vi "Determine Clicked Array Element Index - Determine Array and Scrollbar Properties.vi"(8 "error in (no error)":errorcluster, 10 "Coords of Click":T1, 11 "Array Reference":refnum<vi>) -> (0 "error out":errorcluster, 1 "Scrollbar Properties":T2, 2 "Array Properties":T5, 3 "dup Array Reference":refnum<vi>)   [LabVIEW 2016]
doc: "Determine Clicked Array Element Index - Determine Array and Scrollbar Properties.vi\n\nDescription:\nThis VI determines multiple properties of the array and scrollbars of the array specified by the Array Reference input.\n\nIf no caption has been created for the array of interest, instruct the user how to correct the issue.\n\nInputs:\nArray Reference - Reference to the array to operate on.\n\nCoords of Click - The screen coordinates of the click within the array. These values are used to determine if the click occurred on the selected item.\n\nerror in - Standard error cluster.\n\nOutputs:\ndup Array Reference - Dup reference to the array to operate on.\n\nArray Properties - Cluster containing the array properties of the array specified by the Array Reference input.\n\nScrollbar Properties - Cluster containing the scrollbar properties of the array specified by the Array Reference input.\n\nerror out - standard error cluster.\n\nDeveloped By:\nMark.ridgley\nMark.Ridgley_LabVIEW.Developer@comcast.net"
uses:
  <vilib>/Utility/miscctls.llb/LVBoundsTypeDef.ctl
  <vilib>/Utility/miscctls.llb/LVPositionTypeDef.ctl
  <vilib>/Utility/miscctls.llb/LVPoint32TypeDef.ctl
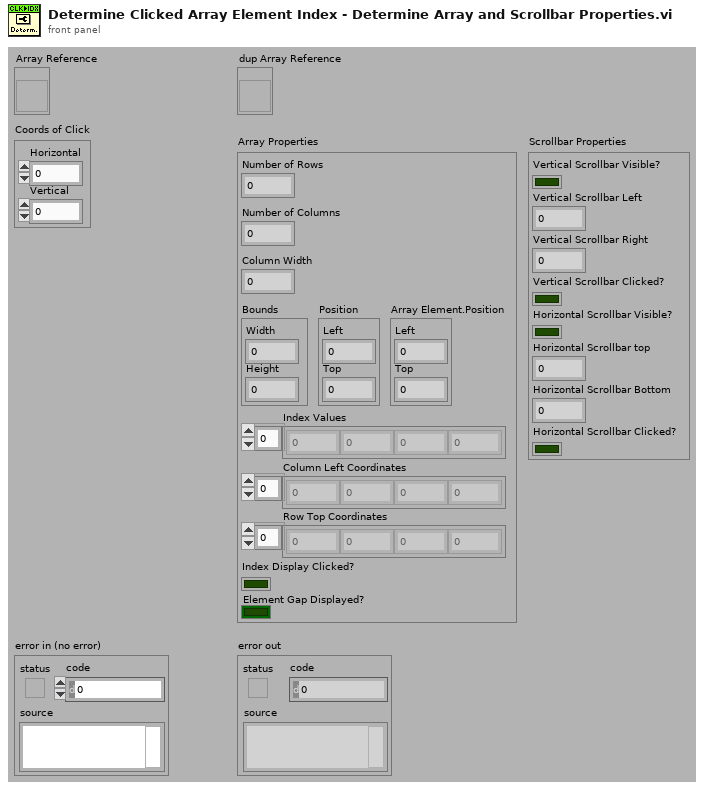
[diagram p1: front panel]
types:
  T1 = typedef "LVPoint32TypeDef.ctl" = cluster{"Horizontal":i32, "Vertical":i32}
  T2 = cluster{"Vertical Scrollbar Visible?":bool, "Vertical Scrollbar Left":i32, "Vertical Scrollbar Right":i32, "Vertical Scrollbar Clicked?":bool, "Horizontal Scrollbar Visible? ":bool, "Horizontal Scrollbar top":i32, "Horizontal Scrollbar Bottom":i32, "Horizontal Scrollbar Clicked?":bool}
  T3 = typedef "LVBoundsTypeDef.ctl" = cluster{"Width":u32, "Height":u32}
  T4 = typedef "LVPositionTypeDef.ctl" = cluster{"Left":i32, "Top":i32}
  T5 = cluster{"Number of Rows":u32, "Number of Columns":u32, "Column Width":u32, "Bounds":T3, "Position":T4, "Array Element.Position":T4, "Index Values":u32[], "Column Left Coordinates":i32[], "Row Top Coordinates":i32[], "Index Display Clicked?":bool, "Element Gap Displayed?":bool}
  T6 = enum16{"Horizontal Scrollbar", "Vertical Scrollbar"}
  T7 = enum16{"Horizontal Scrollbar", "Vertical Scrollbar", "Index Display"}
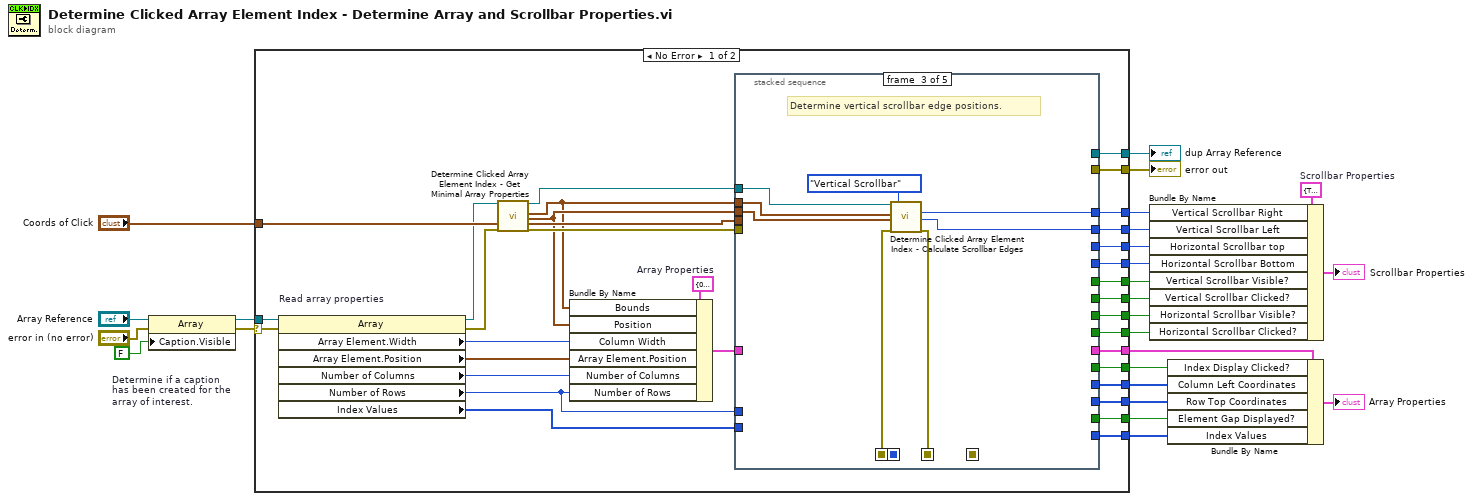
[diagram p0: block diagram]
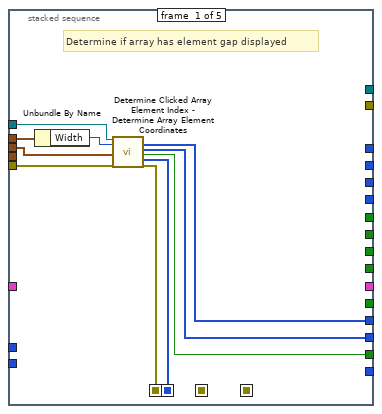
[diagram p2: hidden frame]
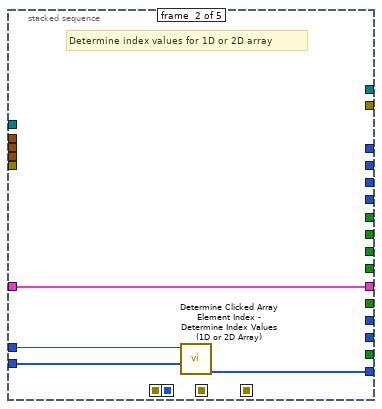
[diagram p3: hidden frame]
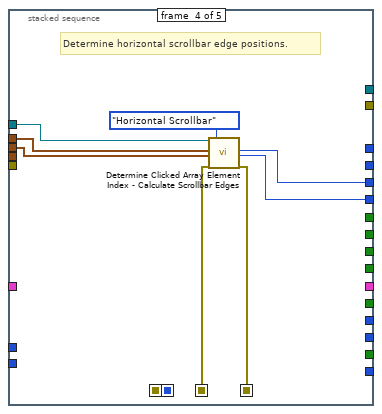
[diagram p4: hidden frame]
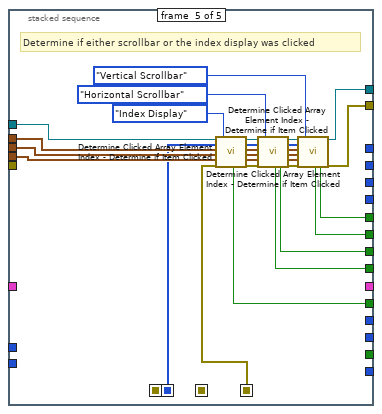
[diagram p5: hidden frame]
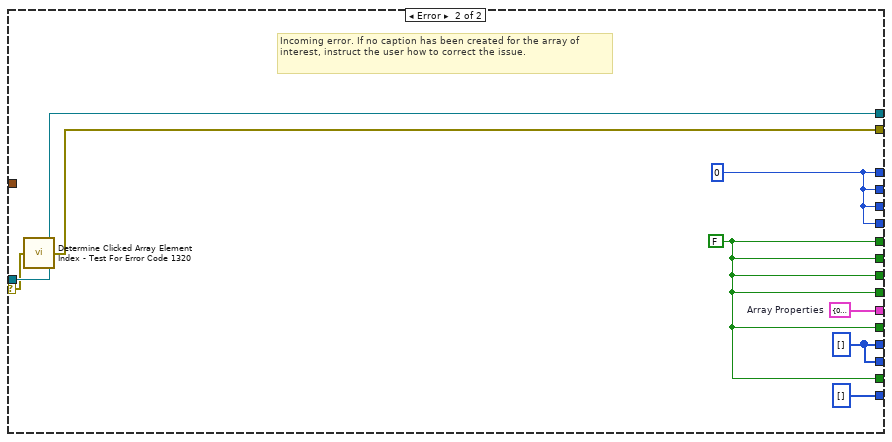
[diagram p6: hidden frame]
diagram:
  w1 = T2 {"Vertical Scrollbar Visible?"=TRUE, "Vertical Scrollbar Left"=0, "Vertical Scrollbar Right"=0, "Vertical Scrollbar Clicked?"=FALSE, "Horizontal Scrollbar Visible? "=TRUE, "Horizontal Scrollbar top"=0, "Horizontal Scrollbar Bottom"=0, "Horizontal Scrollbar Clicked?"=TRUE}  # Scrollbar Properties
  n1 = property on="Determine if a caption has been created for the array of interest." class="Array"(reference="Array Reference", error in="error in (no error)", "Caption.Visible"=FALSE) -> (reference out=w6:refnum<vi>, error out=w7:errorcluster)
  n2 = case shown="No Error" w7 {
    selector: w7 -> [w30 w121]
    tunnel: "Coords of Click" -> [w58 _]
    tunnel: [w57 u32[] [] ("Column Left Coordinates")] -> w23
    tunnel: w6 -> [w56 w124]
    tunnel: [w53 w123] -> w22
    tunnel: [w52 w123] -> w21
    tunnel: [w51 w123] -> w20
    tunnel: [w50 w123] -> w19
    tunnel: [w49 w123] -> w18
    tunnel: [w46 w124] -> w17
    tunnel: [w45 w117] -> w16
    tunnel: [w44 w117] -> w15
    tunnel: [w42 w122] -> w14
    tunnel: [w41 w122] -> w13
    tunnel: [w40 w123] -> w12
    tunnel: [w32 w118] -> w11
    tunnel: [w31 w120] -> w10
    tunnel: [w27 w117] -> w3
    tunnel: [w26 w117] -> w2
    frame No Error {
      w28 = T5 {"Number of Rows"=0, "Number of Columns"=0, "Column Width"=0, "Bounds"={"Width"=0, "Height"=0}, "Position"={"Left"=0, "Top"=0}, "Array Element.Position"={"Left"=0, "Top"=0}, "Index Values"=[], "Column Left Coordinates"=[], "Row Top Coordinates"=[], "Index Display Clicked?"=FALSE, "Element Gap Displayed?"=FALSE}  # Array Properties
      n3 = property on="Read array properties" class="Array"(reference=w56, error in=w30) -> (reference out=w54:refnum<vi>, error out=w55:errorcluster, "Array Element.Width"=w29:u32, "Array Element.Position"=w36:T4, "Number of Columns"=w34:u32, "Number of Rows"=w35:u32, "Index Values"=w37:u32[])
      n4 = call "Determine Clicked Array Element Index - Get Minimal Array Properties.vi"("Array Reference"=w54, "Coords of Click"=w58, "error in (no error)"=w55) -> ("dup Array Reference"=w43:refnum<vi>, "Minimal Array Properties.Bounds"=w38:T3, "Minimal Array Properties.Position"=w39:T4, "dup Coords of Click"=w48:T1, "error out"=w47:errorcluster)  [unwired: 12 in]
      n5 = Bundle By Name(cluster=w28, "Bounds"=w38, "Position"=w39, "Column Width"=w29, "Array Element.Position"=w36, "Number of Columns"=w34, "Number of Rows"=w35) -> (w33:T5)
      n6 = stacked-sequence {
        seq-local: [w64 _ _ _ _] -> [_ _ _ _ w92]
        seq-local: [w61 _ _ _ _] -> [_ _ w77 _ _]
        seq-local: [_ _ w76 _ _] -> [_ _ _ w87 _]
        seq-local: [_ _ _ w86 _] -> [_ _ _ _ w89]
        tunnel: [_ w69 _ _ _] -> w57
        tunnel: w37 -> [_ w72 _ _ _]
        tunnel: [_ _ _ _ w113] -> w53
        tunnel: [_ _ _ _ w112] -> w52
        tunnel: [_ _ _ _ w111] -> w51
        tunnel: [_ _ _ _ w110] -> w50
        tunnel: [_ _ _ _ w109] -> w49
        tunnel: w48 -> [_ _ _ _ w96]
        tunnel: w47 -> [w62 _ _ _ _]
        tunnel: [_ _ _ _ w90] -> w46
        tunnel: [_ _ _ _ w91] -> w31
        tunnel: [_ _ w79 _ _] -> w45
        tunnel: [_ _ w78 _ _] -> w44
        tunnel: w38 -> [w60 _ w75 w83 w95]
        tunnel: w35 -> [_ w71 _ _ _]
        tunnel: w39 -> [w63 _ w74 w82 w94]
        tunnel: w43 -> [w68 _ w80 w88 w93]
        tunnel: [w67 _ _ _ _] -> w42
        tunnel: [w66 _ _ _ _] -> w41
        tunnel: [w65 _ _ _ _] -> w40
        tunnel: w33 -> [_ w70 _ _ _]
        tunnel: [_ w70 _ _ _] -> w32
        tunnel: [_ _ _ w85 _] -> w27
        tunnel: [_ _ _ w84 _] -> w26
        frame #0 {
          # "Determine if array has element gap displayed"
          n7 = Unbundle By Name(w60) -> ("Width"=w59:u32)
          n8 = call "Determine Clicked Array Element Index - Determine Array Element Coordinates.vi"("Array Reference"=w68, "Minimal Array Properties.Bounds.Width"=w59, "Minimal Array Properties.Position"=w63, "error in (no error)"=w62) -> ("Column Left Coordinates"=w67:i32[], "Row Top Coordinates"=w66:i32[], "Array has element gap?"=w65:bool, "Un-gapped left coordinates"=w64:i32[], "error out"=w61:errorcluster)  [unwired: 10 in, 1 out]
        }
        frame #1 {
          # "Determine index values for 1D or 2D array"
          n9 = call "Determine Clicked Array Element Index - Determine Index Values (1D or 2D Array).vi"("Array Property.Index Values"=w72, "Array Property.Number of Rows"=w71) -> ("Index Values (1D or 2D Array)"=w69:u32[])  [unwired: 9 in]
        }
        frame #2 {
          # "Determine vertical scrollbar edge positions."
          n10 = call "Determine Clicked Array Element Index - Calculate Scrollbar Edges.vi"("Array Reference"=w80, "Minimal Array Properties.Bounds"=w75, "Minimal Array Properties.Position"=w74, "error in (no error)"=w77, "Select Item"=T6."Vertical Scrollbar") -> ("Minimum Scrollbar Edge"=w78:i32, "Maximum Scrollbar Edge"=w79:i32, "error out"=w76:errorcluster)  [unwired: 11 in, 1 out]
        }
        frame #3 {
          # "Determine horizontal scrollbar edge positions."
          n11 = call "Determine Clicked Array Element Index - Calculate Scrollbar Edges.vi"("Array Reference"=w88, "Minimal Array Properties.Bounds"=w83, "Minimal Array Properties.Position"=w82, "error in (no error)"=w87, "Select Item"=T6."Horizontal Scrollbar") -> ("Minimum Scrollbar Edge"=w85:i32, "Maximum Scrollbar Edge"=w84:i32, "error out"=w86:errorcluster)  [unwired: 11 in, 1 out]
        }
        frame #4 {
          # "Determine if either scrollbar or the index display was clicked"
          n12 = call "Determine Clicked Array Element Index - Determine if Item Clicked.vi"("Array Reference"=w93, "Un-gapped left coordinates"=w92, "Minimal Array Properties.Bounds"=w95, "Minimal Array Properties.Position"=w94, "Coords of Click"=w96, "error in (no error)"=w89, "Select Item"=T7."Index Display") -> ("Item Clicked?"=w113:bool, "dup Array Reference"=w116:refnum<vi>, "dup Un-gapped left coordinates"=w101:i32[], "dup Minimal Array Properties.Bounds"=w107:T3, "dup Minimal Array Properties.Position"=w103:T4, "dup Coords of Click"=w102:T1, "error out"=w108:errorcluster)  [unwired: 5 in, 1 out]
          n13 = call "Determine Clicked Array Element Index - Determine if Item Clicked.vi"("Array Reference"=w116, "Un-gapped left coordinates"=w101, "Minimal Array Properties.Bounds"=w107, "Minimal Array Properties.Position"=w103, "Coords of Click"=w102, "error in (no error)"=w108, "Select Item"=T7."Horizontal Scrollbar") -> ("Item Clicked?"=w112:bool, "Item Visible?"=w111:bool, "dup Array Reference"=w115:refnum<vi>, "dup Un-gapped left coordinates"=w100:i32[], "dup Minimal Array Properties.Bounds"=w106:T3, "dup Minimal Array Properties.Position"=w105:T4, "dup Coords of Click"=w104:T1, "error out"=w114:errorcluster)  [unwired: 5 in]
          n14 = call "Determine Clicked Array Element Index - Determine if Item Clicked.vi"("Array Reference"=w115, "Un-gapped left coordinates"=w100, "Minimal Array Properties.Bounds"=w106, "Minimal Array Properties.Position"=w105, "Coords of Click"=w104, "error in (no error)"=w114, "Select Item"=T7."Vertical Scrollbar") -> ("Item Clicked?"=w110:bool, "Item Visible?"=w109:bool, "dup Array Reference"=w90:refnum<vi>, "error out"=w91:errorcluster)  [unwired: 5 in, 4 out]
        }
      }
    }
    frame Error {
      w118 = T5 {"Number of Rows"=0, "Number of Columns"=0, "Column Width"=0, "Bounds"={"Width"=0, "Height"=0}, "Position"={"Left"=0, "Top"=0}, "Array Element.Position"={"Left"=0, "Top"=0}, "Index Values"=[], "Column Left Coordinates"=[], "Row Top Coordinates"=[], "Index Display Clicked?"=FALSE, "Element Gap Displayed?"=FALSE}  # Array Properties
      w122 = i32[] [] ("Column Left Coordinates")
      w117 = 0 ("Vertical Scrollbar Right")
      w123 = FALSE ("Item Visible?")
      # "Incoming error. If no caption has been created for the array of interest, instruct the user how to correct the issue."
      n15 = call "Determine Clicked Array Element Index - Test For Error Code 1320.vi"("error in"=w121) -> ("error out"=w120:errorcluster)  [unwired: 14 in]
    }
  }
  "error out" <- w10
  "dup Array Reference" <- w17
  n16 = Bundle By Name(cluster=w1, "Vertical Scrollbar Right"=w15, "Vertical Scrollbar Left"=w16, "Horizontal Scrollbar top"=w3, "Horizontal Scrollbar Bottom"=w2, "Vertical Scrollbar Visible?"=w18, "Vertical Scrollbar Clicked?"=w19, "Horizontal Scrollbar Visible?"=w20, "Horizontal Scrollbar Clicked?"=w21) -> (→"Scrollbar Properties":T2)
  n17 = Bundle By Name(cluster=w11, "Index Display Clicked?"=w22, "Column Left Coordinates"=w14, "Row Top Coordinates"=w13, "Element Gap Displayed?"=w12, "Index Values"=w23) -> (→"Array Properties":T5)
